vi "frame_sel.vi"(8 "正则表达式":string, 10 "帧长":i32, 11 "输入字符串":string) -> (1 "结果":string, 3 "剩余":string)   [LabVIEW 2012]
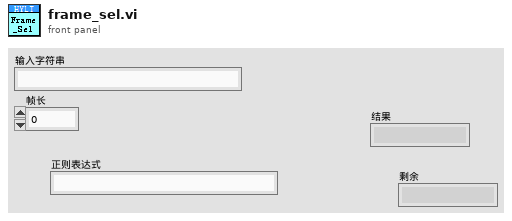
[diagram p1: front panel]
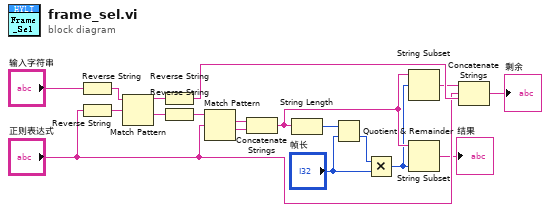
[diagram p0: block diagram]
diagram:
  n1 = Reverse String(1:"输入字符串") -> (0:w15:string)
  n2 = Reverse String(1:"正则表达式") -> (0:w14:string)
  n3 = Match Pattern(string=w15, regular expression=w14) -> (before substring=w18:string, after substring=w17:string)  [unwired: 1 in, 2 out]
  n4 = Reverse String(1:w18) -> (0:w12:string)
  n5 = Reverse String(1:w17) -> (0:w11:string)
  n6 = Match Pattern(string=w11, regular expression="正则表达式") -> (match substring=w9:string, after substring=w8:string)  [unwired: 1 in, 2 out]
  n7 = Concatenate Strings(w9, w8) -> (w3:string)
  n8 = String Length(string=w3) -> (length=w7:i32)
  n9 = Quotient & Remainder(x=w7, y="帧长") -> (floor(x/y)=w6:i32)  [unwired: 1 out]
  n10 = Multiply(x=w6, y="帧长") -> (x*y=w2:i32)
  n11 = String Subset(string=w3, offset (0)=w2) -> (substring=w1:string)  [unwired: 1 in]
  n12 = String Subset(string=w3, length (rest)=w2) -> (substring=→"结果":string)  [unwired: 1 in]
  n13 = Concatenate Strings(w1, "正则表达式", w12) -> (→"剩余":string)
